vi "VectorNav Heading Global.vi"() -> ()   [LabVIEW 2010]
panel:
  out "VectorNav Heading":T1
types:
  T1 = cluster{"Yaw":fxp<+/-,64,32>, "Pitch":fxp<+/-,64,32>, "Roll":fxp<+/-,64,32>}
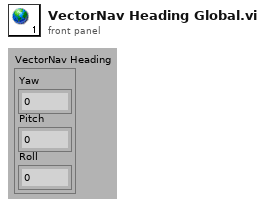
[diagram p1: front panel]
diagram:
